vi "Load Multiple INI Files and Poll for Status Messages.vi"(8 "error in":errorcluster, 11 "List of INI Files":path[](array[path])) -> (0 "error out":errorcluster, 2 "Device Status Messages":T1[](array[typedef]), 3 "Device Configurations":T2[](array[typedef]))   [LabVIEW 2017]
doc: "Loads multiple INI file and retrieves configuration cluster information.\n\nQuerries the device, for the current status."
uses:
  Communications/Typedefs/DTACQ Module Carrier Configuration--Cluster.ctl
  Communications/Typedefs/DTACQ Module Configuration--Cluster.ctl
  Communications/Typedefs/DTACQ Device Type--Enum.ctl
  Status Monitor/Typedefs/Unit Under Test Status--Cluster.ctl
  Status Monitor/Status Monitor Library.lvlib
  Communications/Communications Library.lvlib
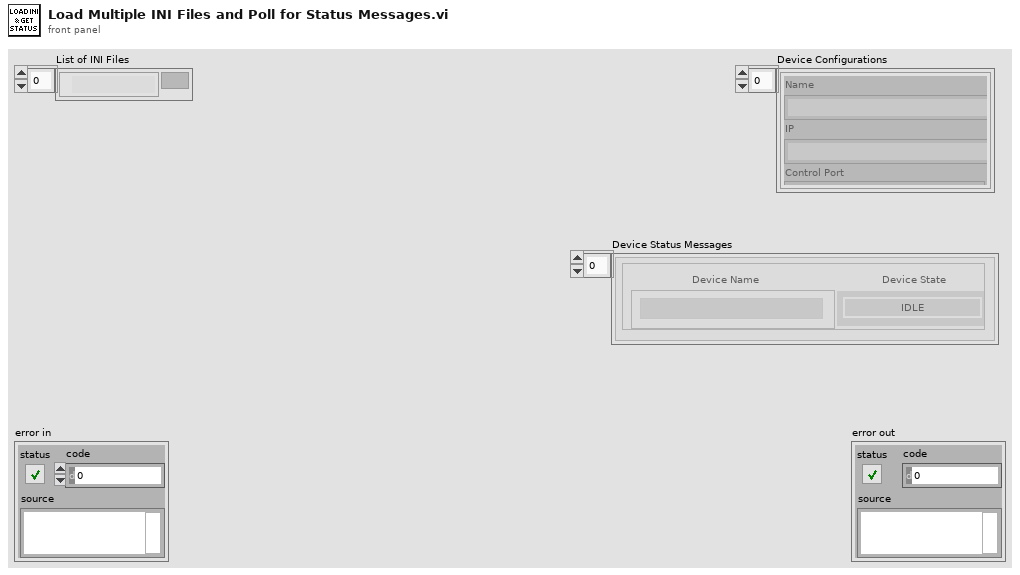
[diagram p1: front panel]
types:
  T1 = typedef "Status Monitor Library.lvlib/Unit Under Test Status--Cluster.ctl" = cluster{"Device State":enum16{"IDLE", "ARM", "RUN_PRE-TRIGGER", "RUN_POST-TRIGGER", "POST_PROCESS", "CLEANUP"}, "Pre-Buffered Samples":i32, "Post-Buffered Samples":i32, "Total Samples":i32, "Demuxing":bool, "Device Name":string}
  T2 = typedef "Communications Library.lvlib/DTACQ Module Carrier Configuration--Cluster.ctl" = cluster{"Name":string, "IP":string, "Control Port":i32, "Timeout (ms)":i32, "Continuous Capture Port (Multiplexed)":i32, "Start HIL Shot Port":i32, "AWG Upload Port (Multiplexed)":i32, "Download Captured Data Port (Multiplexed)":i32, "Module Slots":i32, "Module Configurations":T3[]}
  T3 = typedef "Communications Library.lvlib/DTACQ Module Configuration--Cluster.ctl" = cluster{"Name":string, "Position":string, "Module Type":T4, "Control Port":i32, "Timeout (ms)":i32, "Channels":i32}
  T4 = typedef "Communications Library.lvlib/DTACQ Device Type--Enum.ctl" = enum16{"Carrier", "Analog In Module", "Analog Out Module", "Generic Module"}
  T5 = typedef "Communications Library.lvlib/DTACQ Module Carrier Status.ctl" = cluster{"DTACQ State":T6, "Pre-Trigger Samples":i32, "Post-Trigger Samples":i32, "Total Samples":i32, "Post Processing":bool}
  T6 = typedef "Communications Library.lvlib/DTACQ Status--Enum.ctl" = enum16{"IDLE", "ARM", "RUN_PRE-TRIGGER", "RUN_POST-TRIGGER", "POST_PROCESS", "CLEANUP"}
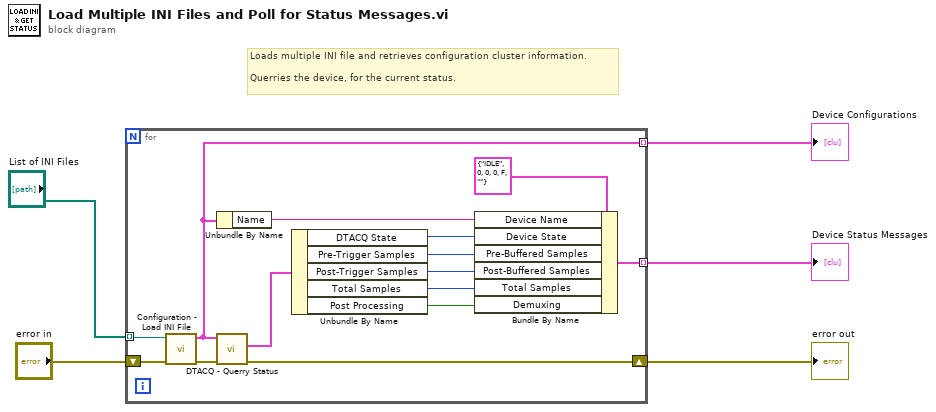
[diagram p0: block diagram]
diagram:
  # "Loads multiple INI file and retrieves configuration cluster information.\n\nQuerries the device, for the current status."
  n1 = for {
    tunnel: "List of INI Files" -> [w19] mode=indexing
    shift-right: [w16] -> w5
    shift-left: "error in" -> [w18]
    tunnel: [w7] -> w2 mode=indexing
    tunnel: [w6] -> w3 mode=indexing
    n2 = call "Configuration - Load INI File.vi"("error in"=w18, "configuration file path"=w19) -> ("error out"=w17:errorcluster, "Carrier Configuration Out"=w6:T2)  [unwired: 8 in]
    n3 = Unbundle By Name(w6) -> ("Name"=w14:string)
    n4 = call "DTACQ - Querry Status.vi"("error in"=w17, "Configuration Cluster"=w6) -> ("error out"=w16:errorcluster, "Module Carrier Status"=w13:T5)  [unwired: 6 in, 2 out]
    n5 = Unbundle By Name(w13) -> ("DTACQ State"=w12:T6, "Pre-Trigger Samples"=w8:i32, "Post-Trigger Samples"=w9:i32, "Total Samples"=w10:i32, "Post Processing"=w11:bool)
    n6 = Bundle By Name(cluster=T1 {"Device State"=enum."IDLE", "Pre-Buffered Samples"=0, "Post-Buffered Samples"=0, "Total Samples"=0, "Demuxing"=FALSE, "Device Name"=""} ("Status Cluster"), "Device Name"=w14, "Device State"=w12, "Pre-Buffered Samples"=w8, "Post-Buffered Samples"=w9, "Total Samples"=w10, "Demuxing"=w11) -> (w7:T1)
  }
  "error out" <- w5
  "Device Configurations" <- w3
  "Device Status Messages" <- w2
